vi "Easy2Acquire.ConvertQuat2Euler.Simple.vi"(10 "GetID":string, 11 "MotionData":dbl[][](array[numeric])) -> (2 "Euler":dbl[][](array[numeric]), 3 "Accel":dbl[][](array[numeric]))   [LabVIEW 2015]
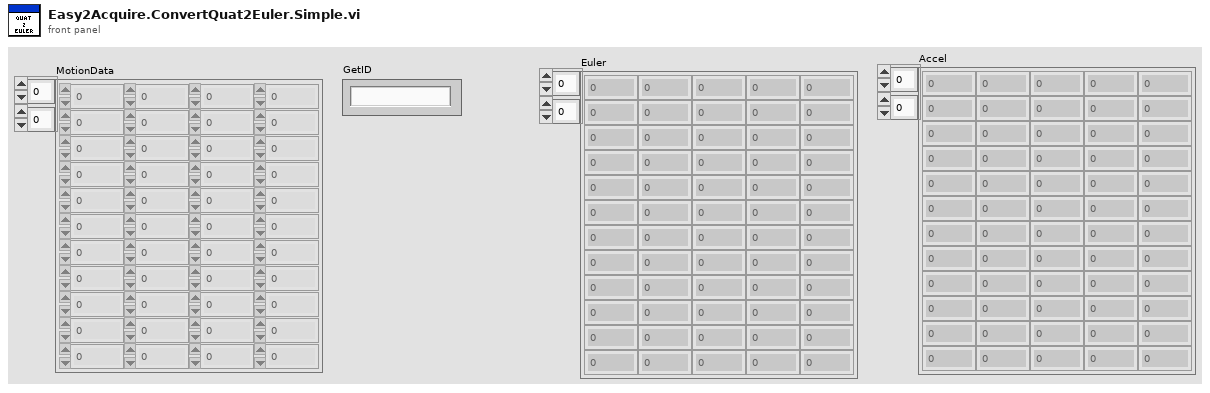
[diagram p1: front panel]
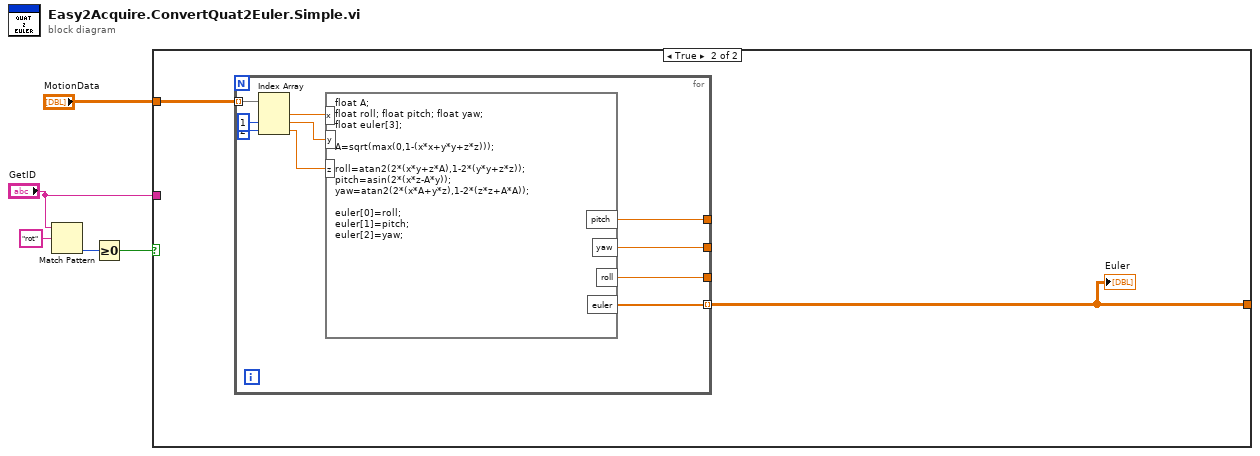
[diagram p0: block diagram]
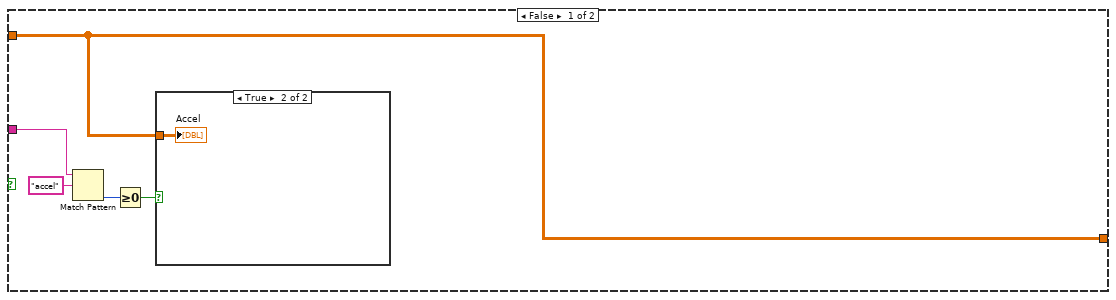
[diagram p2: hidden frame]
diagram:
  n1 = Match Pattern(string="GetID", regular expression="rot") -> (offset past match=w3:i32)  [unwired: 1 in, 3 out]
  n2 = Greater Or Equal To 0?(x=w3) -> (x >= 0?=w4:bool)
  n3 = case shown="True" w4 {
    tunnel: "MotionData" -> [w6 w13]
    tunnel: [w6 w12] -> _
    tunnel: "GetID" -> [w7 _]
    frame False {
      n4 = Match Pattern(string=w7, regular expression="accel") -> (offset past match=w9:i32)  [unwired: 1 in, 3 out]
      n5 = Greater Or Equal To 0?(x=w9) -> (x >= 0?=w8:bool)
      n6 = case shown="True" w8 {
        tunnel: w6 -> [_ w11]
        frame False {
        }
        frame True {
          "Accel" <- w11
        }
      }
    }
    frame True {
      n7 = for {
        tunnel: w13 -> [w23] mode=indexing
        tunnel: [w17] -> w12 mode=indexing
        tunnel: [w16] -> _
        tunnel: [w15] -> _
        tunnel: [w14] -> _
        n8 = Index Array(array=w23, index #2=1 ("index"), index #3=2 ("index")) -> (element #1=w20:dbl, element #2=w19:dbl, element #3=w18:dbl)  [unwired: 1 in]
        n9 = formula code="float A;\nfloat roll; float pitch; float yaw;\nfloat euler[3];\n\nA=sqrt(max(0,1-(x*x+y*y+z*z)));\n\nroll=atan2(2*(x*y+z*A),1-2*(y*y+z*z));\npitch=asin(2*(x*z-A*y));\nyaw=atan2(2*(x*A+y*z),1-2*(z*z+A*A));\n\neuler[0]=roll;\neuler[1]=pitch;\neuler[2]=yaw;"("x"=w20, "y"=w19, "z"=w18) -> ("euler"=w17:dbl[], "roll"=w15:dbl, "pitch"=w16:dbl, "yaw"=w14:dbl)
      }
      "Euler" <- w12
    }
  }
